vi "AB_RW_Project_App_Info.vi"(6 "dataForPrevious in":T1, 7 "action":T2, 8 "error in (no error)":errorcluster, 10 "applicationInfo in":T3, 11 "Object In":T5) -> (0 "error out":errorcluster, 2 "Application info":T3, 3 "Object Out":T5, 4 "dataFromPrevious":T1)   [LabVIEW 2020]
uses:
  <resource>/Framework/Providers/API/ItemRef.ctl
  <vilib>/AppBuilder/RW_Project/AB_RW_Project_App_Data.ctl
  <vilib>/AppBuilder/RW_Project/AB_RW_Project_App_EmbeddedServerConfiguration_Data.ctl
  <vilib>/AppBuilder/RW_Project/AB_RW_Project_PropBag_Action.ctl
  <vilib>/AppBuilder/RW_Project/AB_RW_Project_App_Data_for_Previous.ctl
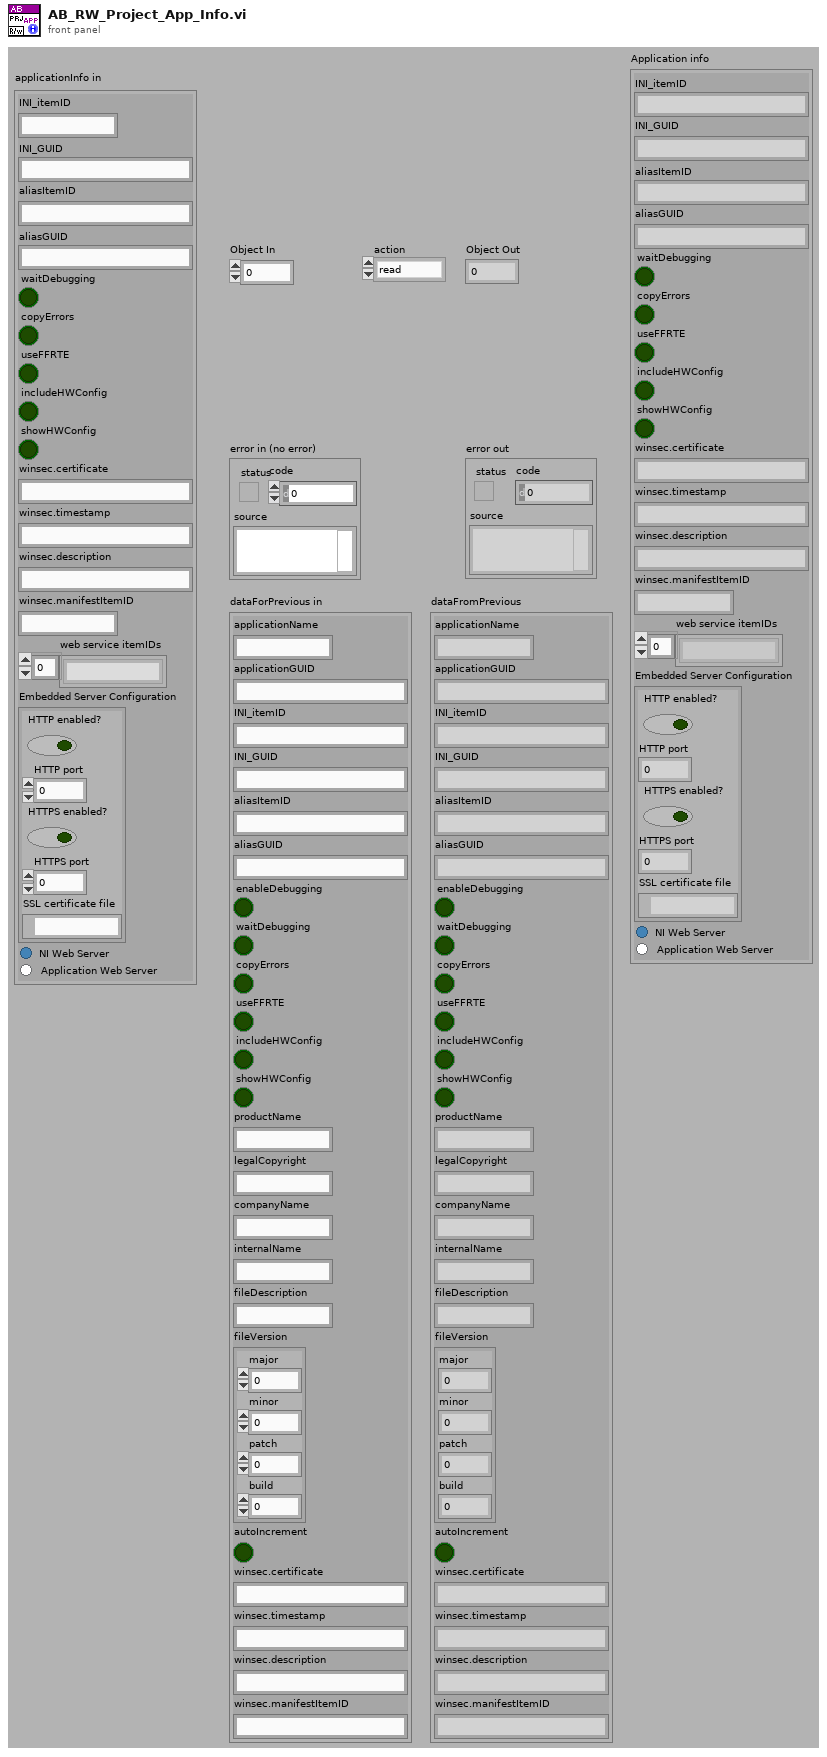
[diagram p1: front panel]
types:
  T1 = typedef "AB_RW_Project_App_Data_for_Previous.ctl" = cluster{"applicationName":string, "applicationGUID":string, "INI_itemID":string, "INI_GUID":string, "aliasItemID":string, "aliasGUID":string, "enableDebugging":bool, "waitDebugging":bool, "copyErrors":bool, "useFFRTE":bool, "includeHWConfig":bool, "showHWConfig":bool, "productName":string, "legalCopyright":string, "companyName":string, "internalName":string, "fileDescription":string, "fileVersion":cluster{"major":u16, "minor":u16, "patch":u16, "build":u16}, "autoIncrement":bool, "winsec.certificate":string, "winsec.timestamp":string, "winsec.description":string, "winsec.manifestItemID":string}
  T2 = typedef "AB_RW_Project_PropBag_Action.ctl" = enum16{"read", "write", "clear", "readPrevious", "writePrevious", "clearPrevious"}
  T3 = typedef "AB_RW_Project_App_Data.ctl" = cluster{"INI_itemID":string, "INI_GUID":string, "aliasItemID":string, "aliasGUID":string, "waitDebugging":bool, "copyErrors":bool, "useFFRTE":bool, "includeHWConfig":bool, "showHWConfig":bool, "winsec.certificate":string, "winsec.timestamp":string, "winsec.description":string, "winsec.manifestItemID":string, "web service itemIDs":string[], "Embedded Server Configuration":T4, "Server Type":enum32{"NI Web Server", "Application Web Server"}}
  T4 = typedef "AB_RW_Project_App_EmbeddedServerConfiguration_Data.ctl" = cluster{"HTTP enabled?":bool, "HTTP port":i32, "HTTPS enabled?":bool, "HTTPS port":i32, "SSL certificate file":path}
  T5 = typedef "ItemRef.ctl" = u64
  T6 = enum32{"NI Web Server", "Application Web Server"}
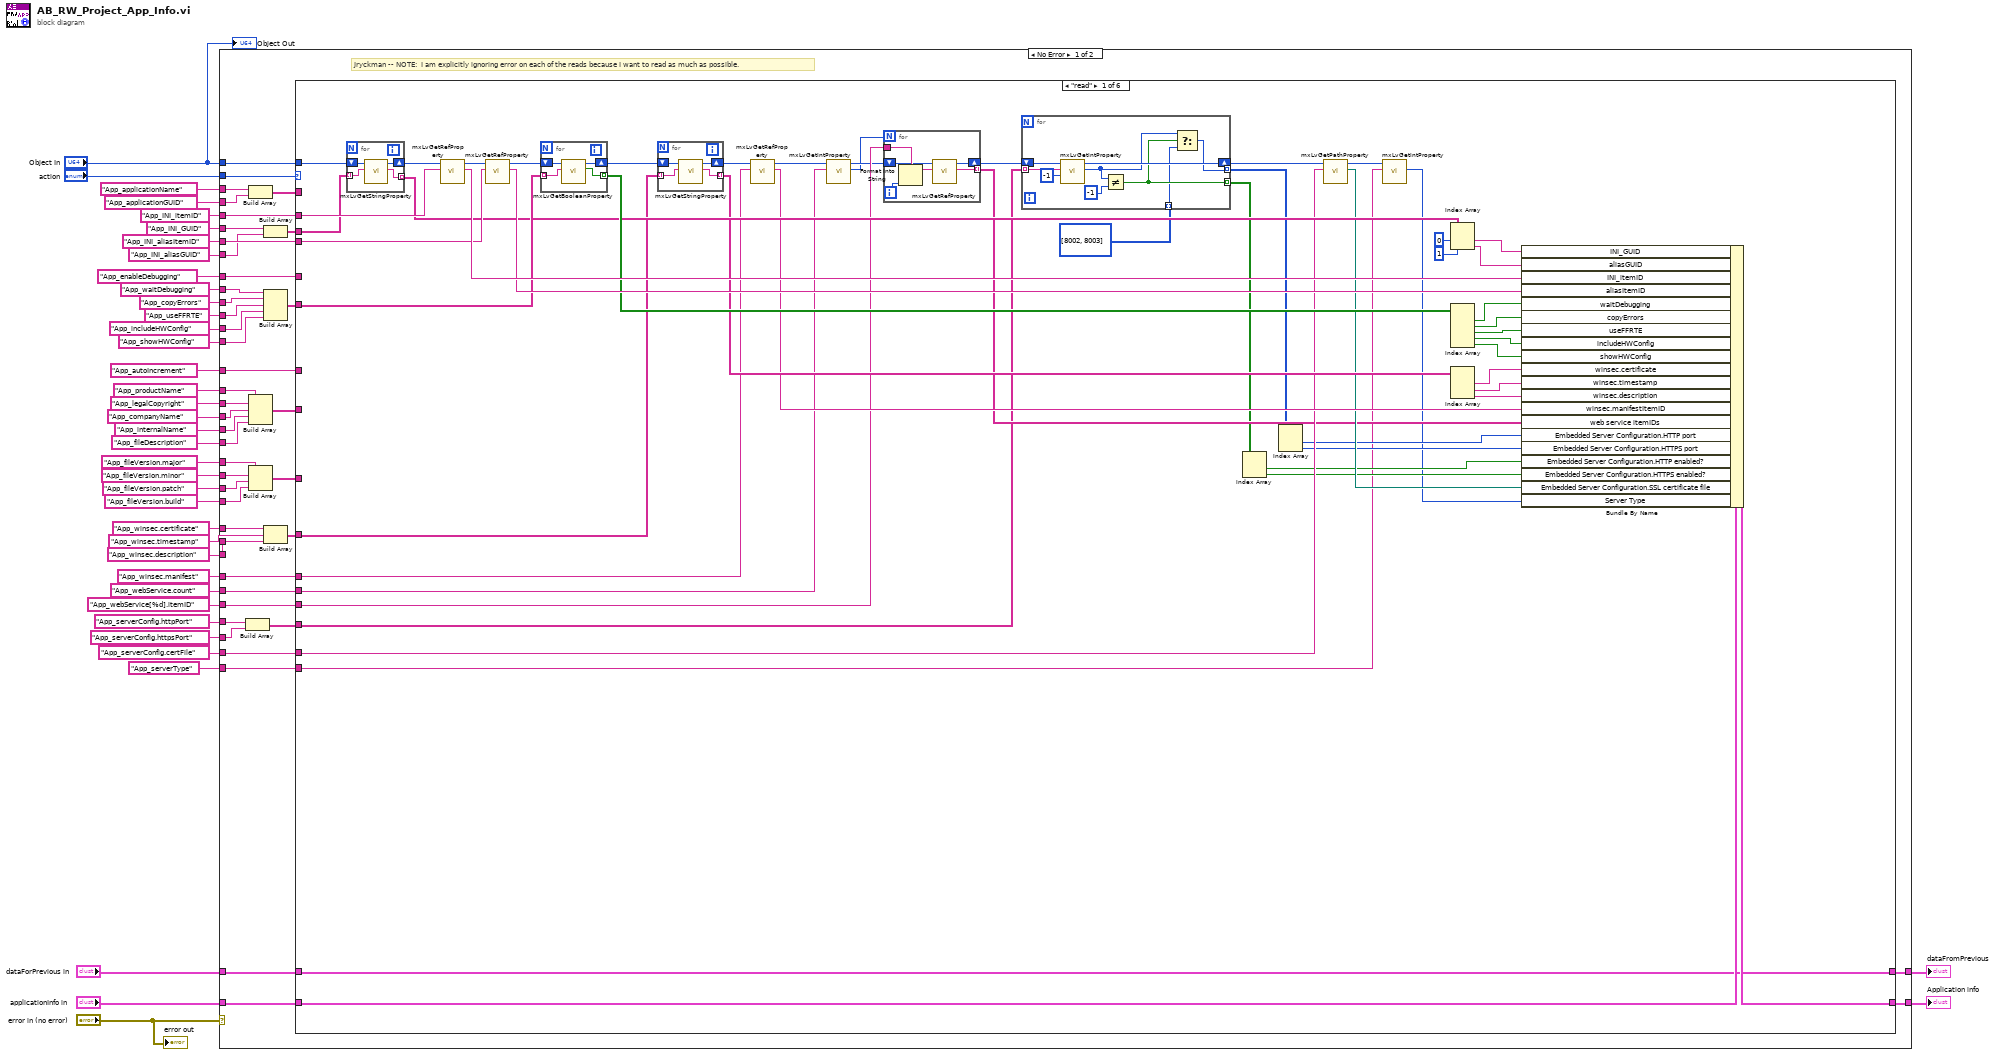
[diagram p0: block diagram]
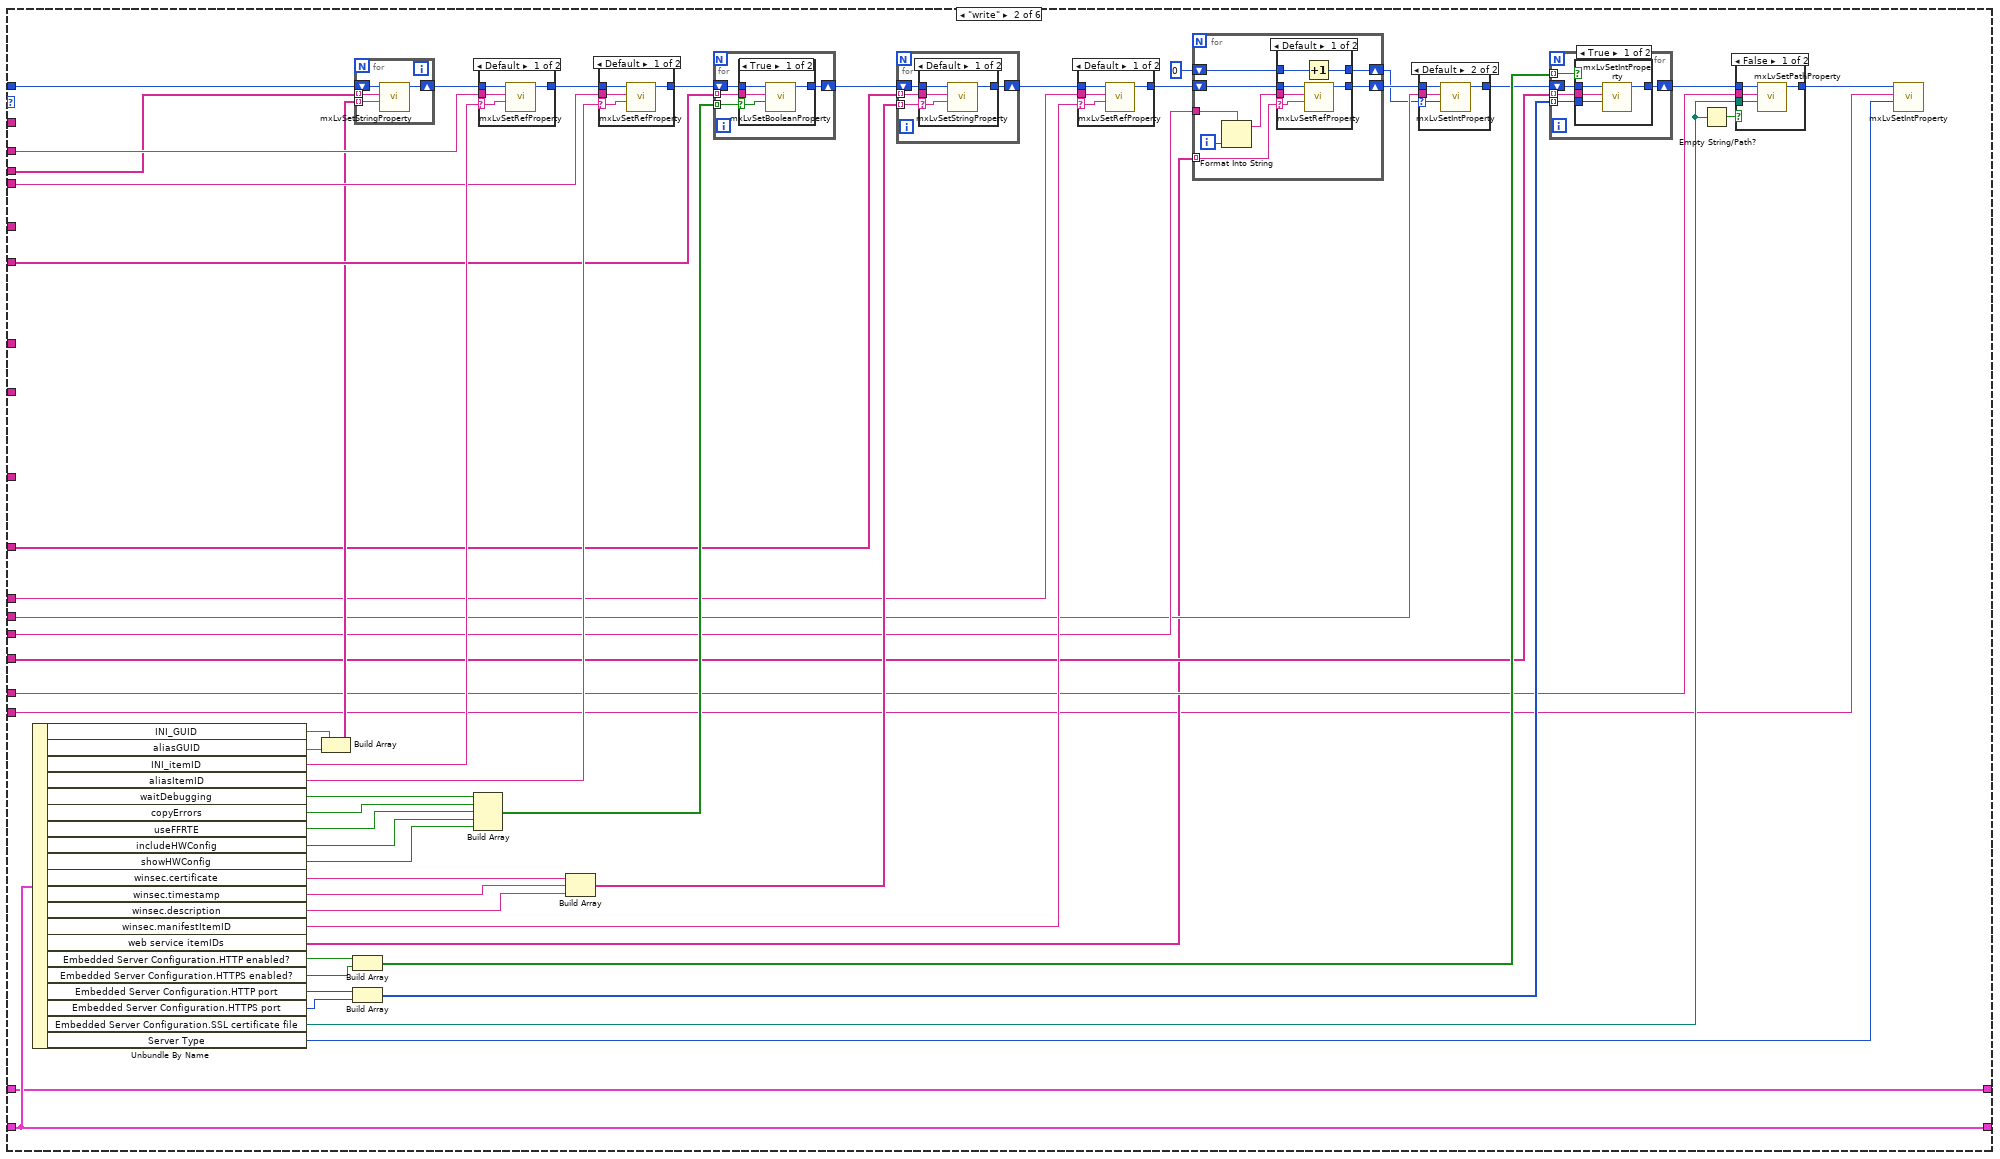
[diagram p2: hidden frame]
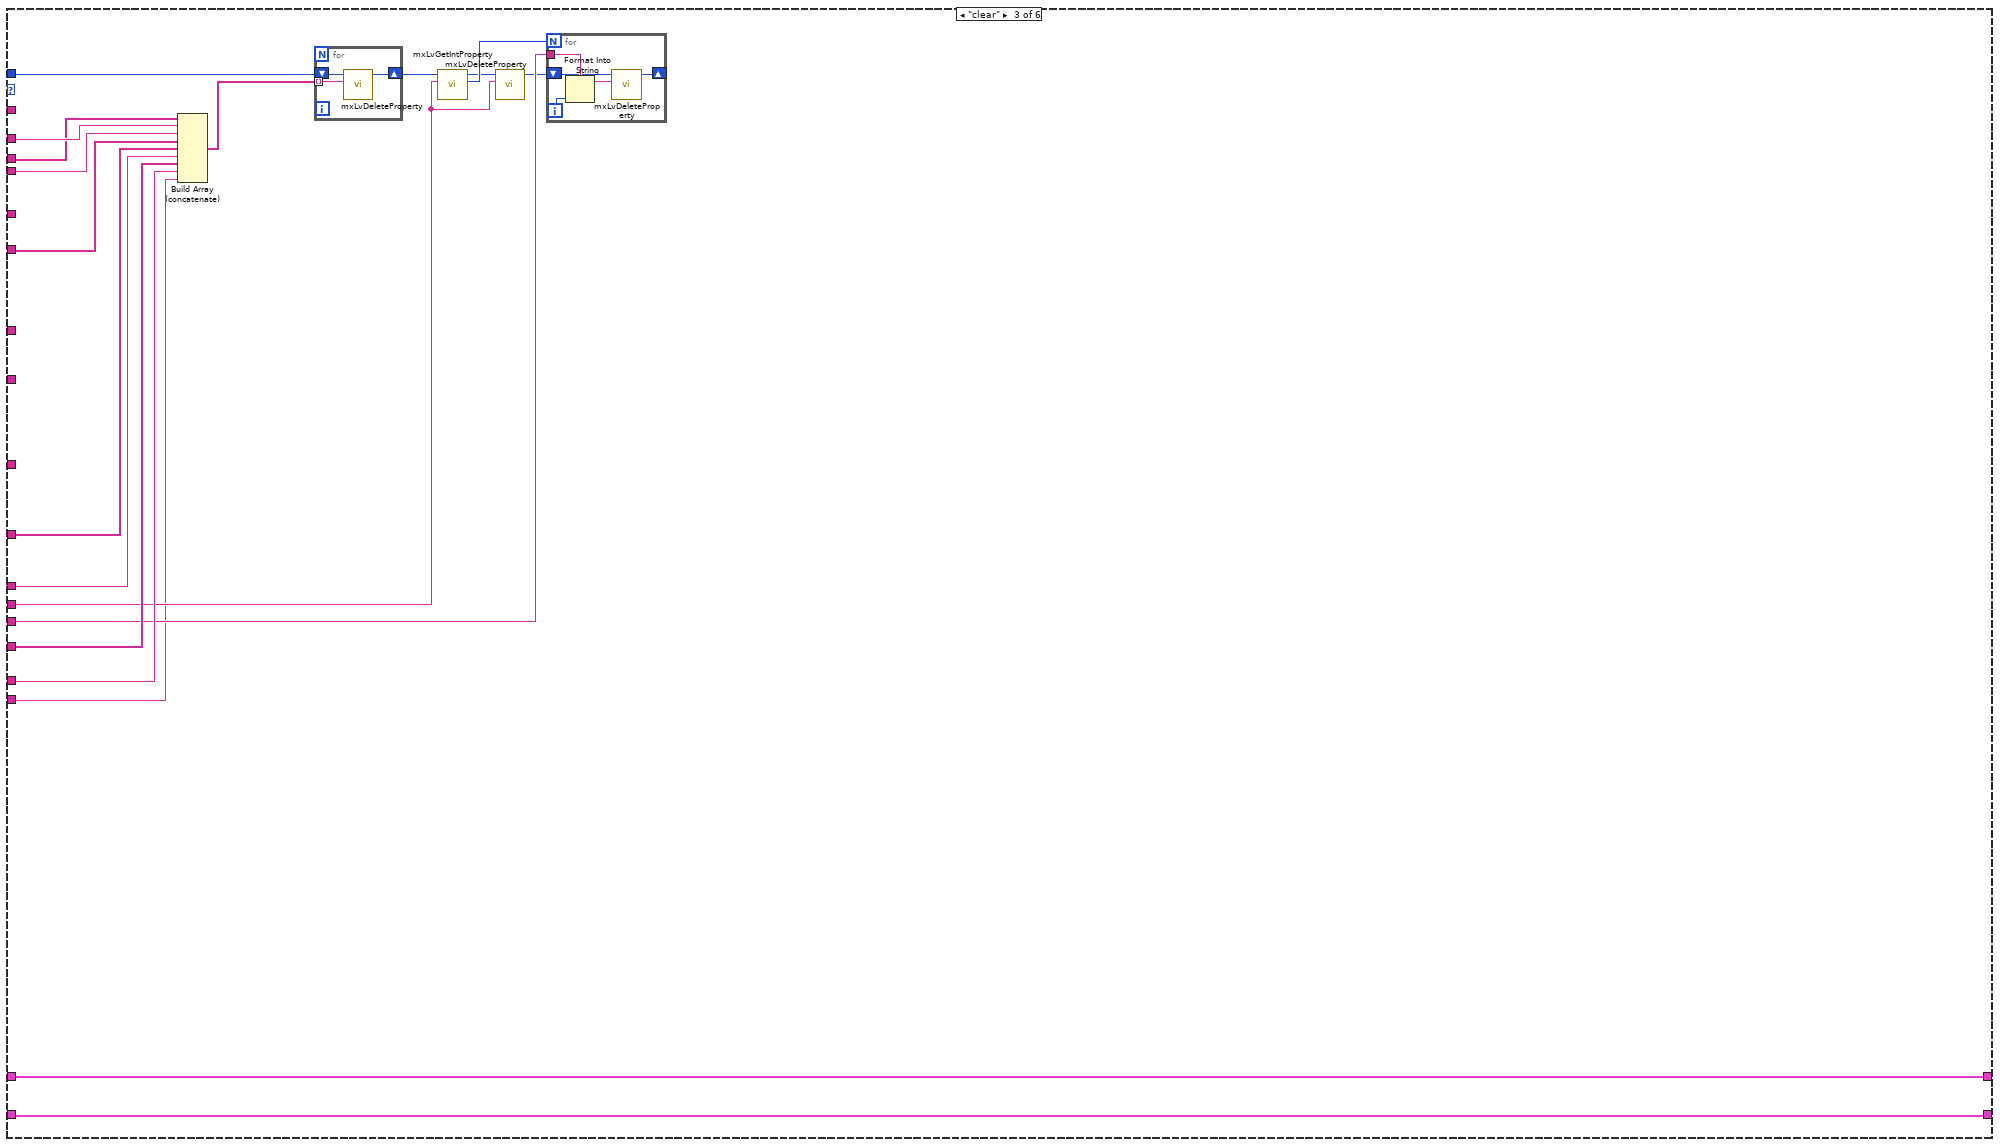
[diagram p12: hidden frame]
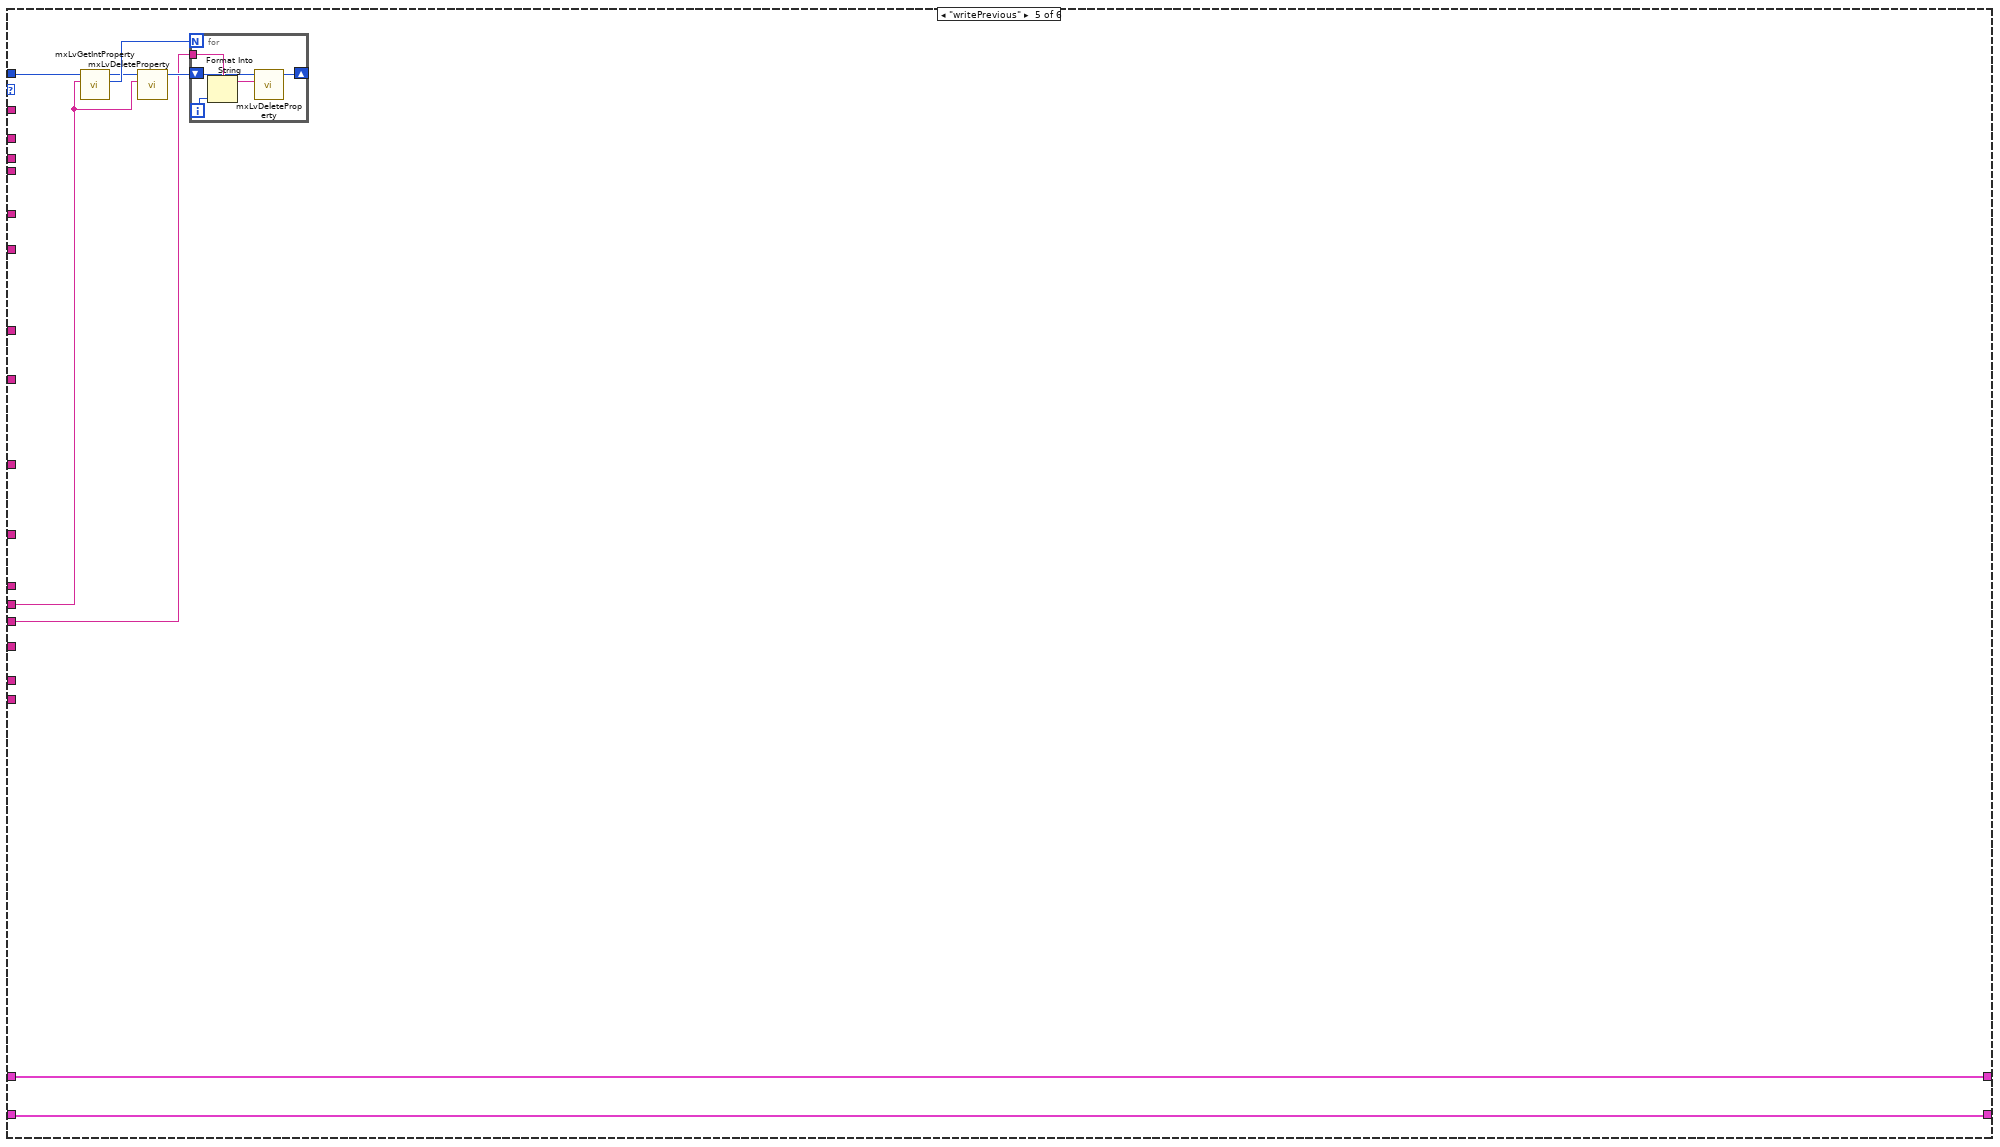
[diagram p14: hidden frame]
diagram:
  n1 = case shown="No Error" "error in (no error)" {
    tunnel: "Object In" -> [w84 _]
    tunnel: [w63 _] -> w37
    tunnel: "applicationInfo in" -> [w69 _]
    tunnel: "App_applicationName" ("Tag") -> [w50 _]
    tunnel: "App_INI_itemID" ("Tag") -> [w83 _]
    tunnel: "App_INI_aliasItemID" ("Tag") -> [w82 _]
    tunnel: "App_enableDebugging" ("Tag") -> [w52 _]
    tunnel: "App_waitDebugging" ("Tag") -> [w81 _]
    tunnel: "App_copyErrors" ("Tag") -> [w80 _]
    tunnel: "App_useFFRTE" ("Tag") -> [w79 _]
    tunnel: "App_includeHWConfig" ("Tag") -> [w78 _]
    tunnel: "App_showHWConfig" ("Tag") -> [w77 _]
    tunnel: "App_productName" ("Tag") -> [w74 _]
    tunnel: "App_legalCopyright" ("Tag") -> [w75 _]
    tunnel: "App_companyName" ("Tag") -> [w73 _]
    tunnel: "App_internalName" ("Tag") -> [w72 _]
    tunnel: "App_fileDescription" ("Tag") -> [w71 _]
    tunnel: "App_fileVersion.major" ("Tag") -> [w67 _]
    tunnel: "App_fileVersion.minor" ("Tag") -> [w68 _]
    tunnel: "App_fileVersion.patch" ("Tag") -> [w66 _]
    tunnel: "App_fileVersion.build" ("Tag") -> [w65 _]
    tunnel: "App_autoIncrement" ("Tag") -> [w51 _]
    tunnel: "action" -> [w62 _]
    tunnel: "App_applicationGUID" ("Tag") -> [w49 _]
    tunnel: "App_INI_GUID" ("Tag") -> [w61 _]
    tunnel: "App_INI_aliasGUID" ("Tag") -> [w60 _]
    tunnel: "App_winsec.certificate" ("Tag") -> [w58 _]
    tunnel: "App_winsec.timestamp" ("Tag") -> [w57 _]
    tunnel: "App_winsec.description" ("Tag") -> [w56 _]
    tunnel: "App_winsec.manifest" ("Tag") -> [w54 _]
    tunnel: "dataForPrevious in" -> [w53 _]
    tunnel: [w47 _] -> w7
    tunnel: "App_webService[%d].itemID" ("Tag") -> [w46 _]
    tunnel: "App_serverConfig.httpPort" ("Tag") -> [w45 _]
    tunnel: "App_serverConfig.httpsPort" ("Tag") -> [w44 _]
    tunnel: "App_serverConfig.certFile" ("Tag") -> [w42 _]
    tunnel: "App_webService.count" ("Tag") -> [w41 _]
    tunnel: "App_serverType" ("Tag") -> [w40 _]
    frame No Error {
      # "Jryckman -- NOTE:  I am explicitly ignoring error on each of the reads because I want to read as much as possible."
      n2 = Build Array(w45, w44) -> (w43:string[])
      n3 = Build Array(w50, w49) -> (w48:string[])
      n4 = Build Array(w74, w75, w73, w72, w71) -> (w70:string[])
      n5 = Build Array(w67, w68, w66, w65) -> (w64:string[])
      n6 = Build Array(w61, w60) -> (w59:string[])
      n7 = Build Array(w81, w80, w79, w78, w77) -> (w76:string[])
      n8 = Build Array(w58, w57, w56) -> (w55:string[])
      n9 = case shown="\"read\"" w62 {
        tunnel: w84 -> [w123 w217 w308 _ w322 _]
        tunnel: w83 -> [w134 w215 w307 _ _ _]
        tunnel: w82 -> [w133 w212 w306 _ _ _]
        tunnel: w76 -> [w131 w203 w305 _ _ _]
        tunnel: w70 -> [_ _ _ _ _ _]
        tunnel: w69 -> [w137 w202 w309 w319 w327 w334]
        tunnel: w64 -> [_ _ _ _ _ _]
        tunnel: [w124 w202 w309 w319 w327 w334] -> w63
        tunnel: w59 -> [w122 w201 w303 _ _ _]
        tunnel: w55 -> [w117 w193 w302 _ _ _]
        tunnel: w54 -> [w110 w192 w301 _ _ _]
        tunnel: w53 -> [w108 w188 w300 w318 w326 w333]
        tunnel: w52 -> [_ _ _ _ _ _]
        tunnel: w51 -> [_ _ _ _ _ _]
        tunnel: w48 -> [_ _ _ _ _ _]
        tunnel: [w108 w188 w300 w318 w326 w333] -> w47
        tunnel: w46 -> [w94 w187 w296 _ w320 _]
        tunnel: w43 -> [w99 w179 w299 _ _ _]
        tunnel: w42 -> [w102 w177 w298 _ _ _]
        tunnel: w41 -> [w90 w172 w293 _ w321 _]
        tunnel: w40 -> [w86 w167 w291 _ _ _]
        frame "read" {
          n10 = for {
            shift-right: [w160] -> w121
            shift-left: w123 -> [w161]
            tunnel: w122 -> [w158] mode=indexing
            tunnel: [w159] -> w120 mode=indexing
            n11 = call <resource>:"mxLvGetStringProperty.vi"("Tag"=w158, "Item"=w161) -> ("Value"=w159:string, "Item"=w160:T5)  [unwired: 1 in, 7 out]
          }
          n12 = call <resource>:"mxLvGetRefProperty.vi"("Tag"=w134, "Item"=w121) -> ("Value"=w136:string, "Item"=w138:T5)  [unwired: 1 in, 7 out]
          n13 = call <resource>:"mxLvGetRefProperty.vi"("Tag"=w133, "Item"=w138) -> ("Value"=w135:string, "Item"=w132:T5)  [unwired: 1 in, 7 out]
          n14 = for {
            shift-right: [w164] -> w109
            shift-left: w132 -> [w165]
            tunnel: w131 -> [w163] mode=indexing
            tunnel: [w162] -> w130 mode=indexing
            n15 = call <resource>:"mxLvGetBooleanProperty.vi"("Tag"=w163, "Item"=w165) -> ("Value"=w162:bool, "Item"=w164:T5)  [unwired: 1 in, 7 out]
          }
          n16 = for {
            shift-right: [w156] -> w112
            shift-left: w109 -> [w157]
            tunnel: w117 -> [w154] mode=indexing
            tunnel: [w155] -> w116 mode=indexing
            n17 = call <resource>:"mxLvGetStringProperty.vi"("Tag"=w154, "Item"=w157) -> ("Value"=w155:string, "Item"=w156:T5)  [unwired: 1 in, 7 out]
          }
          n18 = call <resource>:"mxLvGetRefProperty.vi"("Tag"=w110, "Item"=w112) -> ("Value"=w111:string, "Item"=w93:T5)  [unwired: 1 in, 7 out]
          n19 = call <resource>:"mxLvGetIntProperty.vi"("Tag"=w90, "Item"=w93) -> ("Value"=w91:i32, "Item"=w92:T5)  [unwired: 7 in, 1 out]
          n20 = for {
            N: w91 -> [_]
            tunnel: w94 -> [w153]
            shift-right: [w150] -> w105
            shift-left: w92 -> [w151]
            tunnel: [w149] -> w100 mode=indexing
            i -> [w152]
            n21 = Format Into String(format string=w153, w152) -> (resulting string=w148:string)  [unwired: 2 in, 1 out]
            n22 = call <resource>:"mxLvGetRefProperty.vi"("Tag"=w148, "Item"=w151) -> ("Value"=w149:string, "Item"=w150:T5)  [unwired: 7 in, 1 out]
          }
          n23 = for {
            shift-right: [w146] -> w104
            shift-left: w105 -> [w147]
            tunnel: [w140] -> w89 mode=indexing
            tunnel: w99 -> [w144] mode=indexing
            tunnel: [w142] -> w97 mode=indexing
            tunnel: i32[] [8002, 8003] -> [w139] mode=indexing
            n24 = call <resource>:"mxLvGetIntProperty.vi"("Default Value (0)"=-1, "Tag"=w144, "Item"=w147) -> ("Value"=w141:i32, "Item"=w146:T5)  [unwired: 6 in, 1 out]
            n25 = Not Equal?(x=w141, y=-1 ("Default Value (0)")) -> (x != y?=w142:bool)
            n26 = Select(t=w141, s=w142, f=w139) -> (s? t:f=w140:i32)
          }
          n27 = Index Array(array=w97) -> (element #1=w96:bool, element #2=w95:bool)  [unwired: 2 in]
          n28 = Index Array(array=w89) -> (element #1=w98:i32, element #2=w101:i32)  [unwired: 2 in]
          n29 = call <resource>:"mxLvGetPathProperty.vi"("Tag"=w102, "Item"=w104) -> ("Path"=w103:path, "Item"=w87:T5)  [unwired: 7 in, 1 out]
          n30 = call <resource>:"mxLvGetIntProperty.vi"("Tag"=w86, "Item"=w87) -> ("Value"=w85:i32)  [unwired: 7 in, 2 out]
          n31 = Index Array(array=w120, index #1=0 ("index"), index #2=1 ("index")) -> (element #1=w119:string, element #2=w118:string)
          n32 = Index Array(array=w130) -> (element #1=w129:bool, element #2=w128:bool, element #3=w127:bool, element #4=w126:bool, element #5=w125:bool)  [unwired: 5 in]
          n33 = Index Array(array=w116) -> (element #1=w115:string, element #2=w114:string, element #3=w113:string)  [unwired: 3 in]
          n34 = Bundle By Name(cluster=w137, "INI_GUID"=w119, "aliasGUID"=w118, "INI_itemID"=w136, "aliasItemID"=w135, "waitDebugging"=w129, "copyErrors"=w128, "useFFRTE"=w127, "includeHWConfig"=w126, "showHWConfig"=w125, "winsec.certificate"=w115, "winsec.timestamp"=w114, "winsec.description"=w113, "winsec.manifestItemID"=w111, "web service itemIDs"=w100, "Embedded Server Configuration.HTTP port"=w98, "Embedded Server Configuration.HTTPS port"=w101, "Embedded Server Configuration.HTTP enabled?"=w96, "Embedded Server Configuration.HTTPS enabled?"=w95, "Embedded Server Configuration.SSL certificate file"=w103, "Server Type"=w85) -> (w124:T3)
        }
        frame "write" {
          n35 = Unbundle By Name(w202) -> ("INI_GUID"=w198:string, "aliasGUID"=w200:string, "INI_itemID"=w214:string, "aliasItemID"=w211:string, "waitDebugging"=w209:bool, "copyErrors"=w208:bool, "useFFRTE"=w207:bool, "includeHWConfig"=w206:bool, "showHWConfig"=w205:bool, "winsec.certificate"=w197:string, "winsec.timestamp"=w196:string, "winsec.description"=w195:string, "winsec.manifestItemID"=w190:string, "web service itemIDs"=w171:string[], "Embedded Server Configuration.HTTP enabled?"=w185:bool, "Embedded Server Configuration.HTTPS enabled?"=w184:bool, "Embedded Server Configuration.HTTP port"=w183:i32, "Embedded Server Configuration.HTTPS port"=w182:i32, "Embedded Server Configuration.SSL certificate file"=w176:path, "Server Type"=w166:T6)
          n36 = Build Array(w198, w200) -> (w199:string[])
          n37 = Build Array(w185, w184) -> (w181:bool[])
          n38 = Build Array(w183, w182) -> (w180:i32[])
          n39 = for {
            tunnel: w201 -> [w269] mode=indexing
            tunnel: w199 -> [w268] mode=indexing
            shift-right: [w270] -> w216
            shift-left: w217 -> [w271]
            n40 = call <resource>:"mxLvSetStringProperty.vi"("Value (\"\")"=w268, "Tag"=w269, "Item"=w271) -> ("Item"=w270:T5)  [unwired: 2 in, 6 out]
          }
          n41 = Build Array(w209, w208, w207, w206, w205) -> (w204:bool[])
          n42 = case shown="Default" w214 {
            selector: w214 -> [w287 _]
            tunnel: w216 -> [w289 w290]
            tunnel: w215 -> [w288 _]
            tunnel: [w286 w290] -> w213
            frame Default {
              n43 = call <resource>:"mxLvSetRefProperty.vi"("Value (\"\")"=w287, "Tag"=w288, "Item"=w289) -> ("Item"=w286:T5)  [unwired: 2 in, 6 out]
            }
            frame "" {
            }
          }
          n44 = Build Array(w197, w196, w195) -> (w194:string[])
          n45 = case shown="Default" w211 {
            selector: w211 -> [w282 _]
            tunnel: w213 -> [w284 w285]
            tunnel: w212 -> [w283 _]
            tunnel: [w281 w285] -> w210
            frame Default {
              n46 = call <resource>:"mxLvSetRefProperty.vi"("Value (\"\")"=w282, "Tag"=w283, "Item"=w284) -> ("Item"=w281:T5)  [unwired: 2 in, 6 out]
            }
            frame "" {
            }
          }
          n47 = for {
            tunnel: w204 -> [w274] mode=indexing
            shift-right: [w273] -> w189
            shift-left: w210 -> [w275]
            tunnel: w203 -> [w272] mode=indexing
            n48 = case shown="True" w274 {
              selector: w274 -> [w278 _]
              tunnel: w275 -> [w279 w280]
              tunnel: w272 -> [w276 _]
              tunnel: [w277 w280] -> w273
              frame True {
                n49 = call <resource>:"mxLvSetBooleanProperty.vi"("Value (F)"=w278, "Tag"=w276, "Item"=w279) -> ("Item"=w277:T5)  [unwired: 2 in, 6 out]
              }
              frame False {
              }
            }
          }
          n50 = for {
            tunnel: w194 -> [w261] mode=indexing
            shift-right: [w260] -> w191
            shift-left: w189 -> [w262]
            tunnel: w193 -> [w259] mode=indexing
            n51 = case shown="Default" w261 {
              selector: w261 -> [w264 _]
              tunnel: w262 -> [w266 w267]
              tunnel: w259 -> [w263 _]
              tunnel: [w265 w267] -> w260
              frame Default {
                n52 = call <resource>:"mxLvSetStringProperty.vi"("Value (\"\")"=w264, "Tag"=w263, "Item"=w266) -> ("Item"=w265:T5)  [unwired: 2 in, 6 out]
              }
              frame "" {
              }
            }
          }
          n53 = case shown="Default" w190 {
            selector: w190 -> [w255 _]
            tunnel: w191 -> [w257 w258]
            tunnel: w192 -> [w256 _]
            tunnel: [w254 w258] -> w186
            frame Default {
              n54 = call <resource>:"mxLvSetRefProperty.vi"("Value (\"\")"=w255, "Tag"=w256, "Item"=w257) -> ("Item"=w254:T5)  [unwired: 2 in, 6 out]
            }
            frame "" {
            }
          }
          n55 = for {
            tunnel: w187 -> [w245]
            tunnel: w171 -> [w243] mode=indexing
            shift-right: [w241] -> w174
            shift-left: w186 -> [w242]
            shift-right: [w238] -> w169
            shift-left: 0 -> [w239]
            i -> [w244]
            n56 = Format Into String(format string=w245, w244) -> (resulting string=w240:string)  [unwired: 2 in, 1 out]
            n57 = case shown="Default" w243 {
              selector: w243 -> [w246 _]
              tunnel: w242 -> [w249 w253]
              tunnel: w240 -> [w247 _]
              tunnel: [w248 w253] -> w241
              tunnel: w239 -> [w251 w252]
              tunnel: [w250 w252] -> w238
              frame Default {
                n58 = Increment(x=w251) -> (x+1=w250:i32)
                n59 = call <resource>:"mxLvSetRefProperty.vi"("Value (\"\")"=w246, "Tag"=w247, "Item"=w249) -> ("Item"=w248:T5)  [unwired: 7 in, 1 out]
              }
              frame "" {
              }
            }
          }
          n60 = case shown="Default" w169 {
            selector: w169 -> [_ w220]
            tunnel: w174 -> [w218 w222]
            tunnel: [w218 w221] -> w173
            tunnel: w172 -> [_ w219]
            frame 0 {
            }
            frame Default {
              n61 = call <resource>:"mxLvSetIntProperty.vi"("Value (0)"=w220, "Tag"=w219, "Item"=w222) -> ("Item"=w221:T5)  [unwired: 7 in, 1 out]
            }
          }
          n62 = for {
            tunnel: w181 -> [w231] mode=indexing
            shift-right: [w230] -> w178
            shift-left: w173 -> [w232]
            tunnel: w180 -> [w229] mode=indexing
            tunnel: w179 -> [w228] mode=indexing
            n63 = case shown="True" w231 {
              tunnel: w232 -> [w236 w237]
              tunnel: w229 -> [w234 _]
              tunnel: [w235 w237] -> w230
              tunnel: w228 -> [w233 _]
              frame True {
                n64 = call <resource>:"mxLvSetIntProperty.vi"("Value (0)"=w234, "Tag"=w233, "Item"=w236) -> ("Item"=w235:T5)  [unwired: 7 in, 1 out]
              }
              frame False {
              }
            }
          }
          n65 = Empty String/Path?(string/path=w176) -> (empty?=w175:bool)
          n66 = case shown="False" w175 {
            tunnel: w178 -> [w226 w227]
            tunnel: w177 -> [w225 _]
            tunnel: w176 -> [w224 _]
            tunnel: [w223 w227] -> w168
            frame False {
              n67 = call <resource>:"mxLvSetPathProperty.vi"("Path"=w224, "Tag"=w225, "Item"=w226) -> ("Item"=w223:T5)  [unwired: 7 in, 1 out]
            }
            frame True {
            }
          }
          n68 = call <resource>:"mxLvSetIntProperty.vi"("Value (0)"=w166, "Tag"=w167, "Item"=w168) -> ()  [unwired: 7 in, 2 out]
        }
        frame "clear" {
          n69 = Build Array (concatenate)(w303, w307, w306, w305, w302, w301, w299, w298, w291) -> (w304:string[])
          n70 = for {
            tunnel: w304 -> [w316] mode=indexing
            shift-right: [w315] -> w292
            shift-left: w308 -> [w317]
            n71 = call <resource>:"mxLvDeleteProperty.vi"("Tag"=w316, "Item"=w317) -> ("Item"=w315:T5)  [unwired: 1 in, 8 out]
          }
          n72 = call <resource>:"mxLvGetIntProperty.vi"("Tag"=w293, "Item"=w292) -> ("Value"=w297:i32, "Item"=w295:T5)  [unwired: 7 in, 1 out]
          n73 = call <resource>:"mxLvDeleteProperty.vi"("Tag"=w293, "Item"=w295) -> ("Item"=w294:T5)  [unwired: 1 in, 8 out]
          n74 = for {
            N: w297 -> [_]
            tunnel: w296 -> [w314]
            shift-right: [w310] -> _
            shift-left: w294 -> [w312]
            i -> [w313]
            n75 = Format Into String(format string=w314, w313) -> (resulting string=w311:string)  [unwired: 2 in, 1 out]
            n76 = call <resource>:"mxLvDeleteProperty.vi"("Tag"=w311, "Item"=w312) -> ("Item"=w310:T5)  [unwired: 1 in, 8 out]
          }
        }
        frame "readPrevious" {
        }
        frame "writePrevious" {
          n77 = call <resource>:"mxLvGetIntProperty.vi"("Tag"=w321, "Item"=w322) -> ("Value"=w325:i32, "Item"=w324:T5)  [unwired: 7 in, 1 out]
          n78 = call <resource>:"mxLvDeleteProperty.vi"("Tag"=w321, "Item"=w324) -> ("Item"=w323:T5)  [unwired: 1 in, 8 out]
          n79 = for {
            N: w325 -> [_]
            tunnel: w320 -> [w332]
            shift-right: [w328] -> _
            shift-left: w323 -> [w330]
            i -> [w331]
            n80 = Format Into String(format string=w332, w331) -> (resulting string=w329:string)  [unwired: 2 in, 1 out]
            n81 = call <resource>:"mxLvDeleteProperty.vi"("Tag"=w329, "Item"=w330) -> ("Item"=w328:T5)  [unwired: 1 in, 8 out]
          }
        }
        frame "clearPrevious" {
        }
      }
    }
    frame Error {
    }
  }
  "Application info" <- w37
  "dataFromPrevious" <- w7
  "Object Out" <- "Object In"
  "error out" <- "error in (no error)"
